vi "SVL Peak Sound Level (N Ch).vi"(6 "restart averaging (F)":bool, 8 "error in (no error)":errorcluster, 11 "scaled signals [EU]":waveform(dbl)[](array[waveform])) -> (0 "error out":errorcluster, 2 "unit labels":string[](array[string]), 3 "peak sound levels [dB pk EU]":dbl[](array[numeric]) format="%.2f")   [LabVIEW 2017, in "SoundVib_SoundLevel.lvlib"]
doc: "Computes the peak sound level of <B>scaled signal [EU]</B>. <B>scaled signal [EU]</B> should have a zero DC component. You can attenuate the DC component with hardware AC-coupling filters and with software high-pass filters. The peak sound level is the maximum of the absolute values of all measured values. Wire data to the <B>scaled signal [EU]</B> input to determine the polymorphic instance to use or manually select the instance."
uses:
  <vilib>/addons/Sound and Vibration/svt_Level/SoundVib_SoundLevel.lvlib
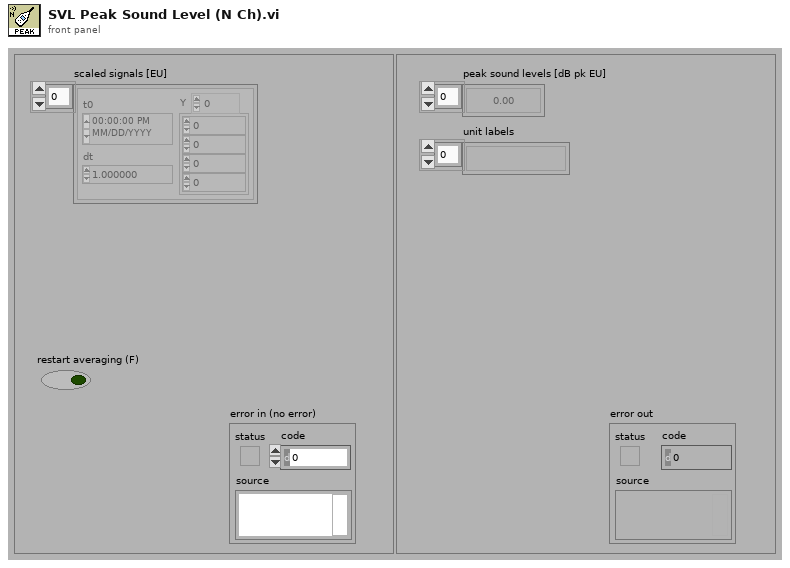
[diagram p1: front panel]
types:
  T1 = enum16{"RMS", "Running RMS", "Exp avg  ", "Dec exp avg ", "Peak", "Crest"}
  T2 = enum16{"Reset filter", "Restart averaging", "Continue processing"}
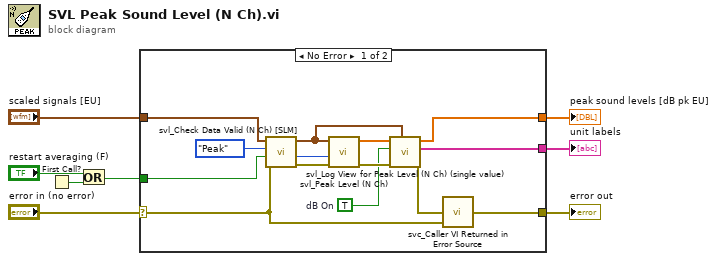
[diagram p0: block diagram]
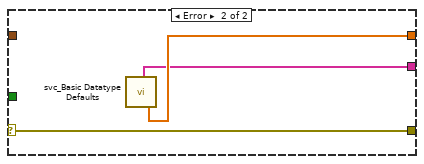
[diagram p2: hidden frame]
diagram:
  n1 = First Call?() -> (First Call?: T/F=w3:bool)
  n2 = Or(x="restart averaging (F)", y=w3) -> (x .or. y?=w2:bool)
  n3 = case shown="No Error" "error in (no error)" {
    tunnel: [w20 w23] -> w6
    tunnel: [w19 w24] -> w5
    tunnel: "scaled signals [EU]" -> [w11 _]
    tunnel: w2 -> [w16 _]
    selector: "error in (no error)" -> [w9 w25]
    tunnel: [w14 w25] -> w7
    frame No Error {
      w12 = TRUE  # dB On
      n4 = call <vilib>:"svl_Check Data Valid (N Ch) [SLM].vi"("error in (no error)"=w9, "restart averaging (F)"=w16, "level analysis"=T1."Peak" ("Level Analysis"), "scaled signals [EU]"=w11) -> ("error out"=w17:errorcluster, "processing state"=w15:T2, "dup scaled signals [EU]"=w10:waveform(dbl)[])  [unwired: 5 in]
      n5 = call <vilib>:"svl_Peak Level (N Ch).vi"("error in (no error)"=w17, "processing state"=w15, "scaled signals [EU]"=w10) -> ("error out"=w21:errorcluster, "peak levels"=w18:dbl[])  [unwired: 7 in]
      n6 = call <vilib>:"svl_Log View for Peak Level (N Ch) (single value).vi"("scaled signals [EU]"=w10, "error in (no error)"=w21, "dB On (T)"=w12, "peak levels [EU]"=w18) -> ("error out"=w22:errorcluster, "unit label [ ]"=w20:string[], "peak levels [EU]"=w19:dbl[])  [unwired: 5 in]
      n7 = call <vilib>:"svc_Caller VI Returned in Error Source.vi"("warning input to caller"=w9, "error in (no error)"=w22) -> ("error out"=w14:errorcluster)  [unwired: 3 in]
    }
    frame Error {
      n8 = call <vilib>:"svc_Basic Datatype Defaults.vi"() -> ("empty array of strings"=w23:string[], "empty array of DBL"=w24:dbl[])  [unwired: 7 in, 11 out]
    }
  }
  "peak sound levels [dB pk EU]" <- w5
  "unit labels" <- w6
  "error out" <- w7
